vi "Update Array.vi"() -> ()   [LabVIEW 2013]
uses:
  Lockins.ctl
  Lockin.ctl
panel:
  in  "OSC used":i32
  in  "OSC Configuration":T1(array[cluster])
  out "Array":cluster{"Y":dbl[], "Y":dbl[]}[][](array[cluster])
  in  "Reset":bool=TRUE
  in  "Temperature":dbl
  in  "Lockins":T2 items=["Lock-in #1", "Lock-in #2", "Lock-in #3", "Lock-in #4"]
  in  "Results":dbl[][](array[numeric])
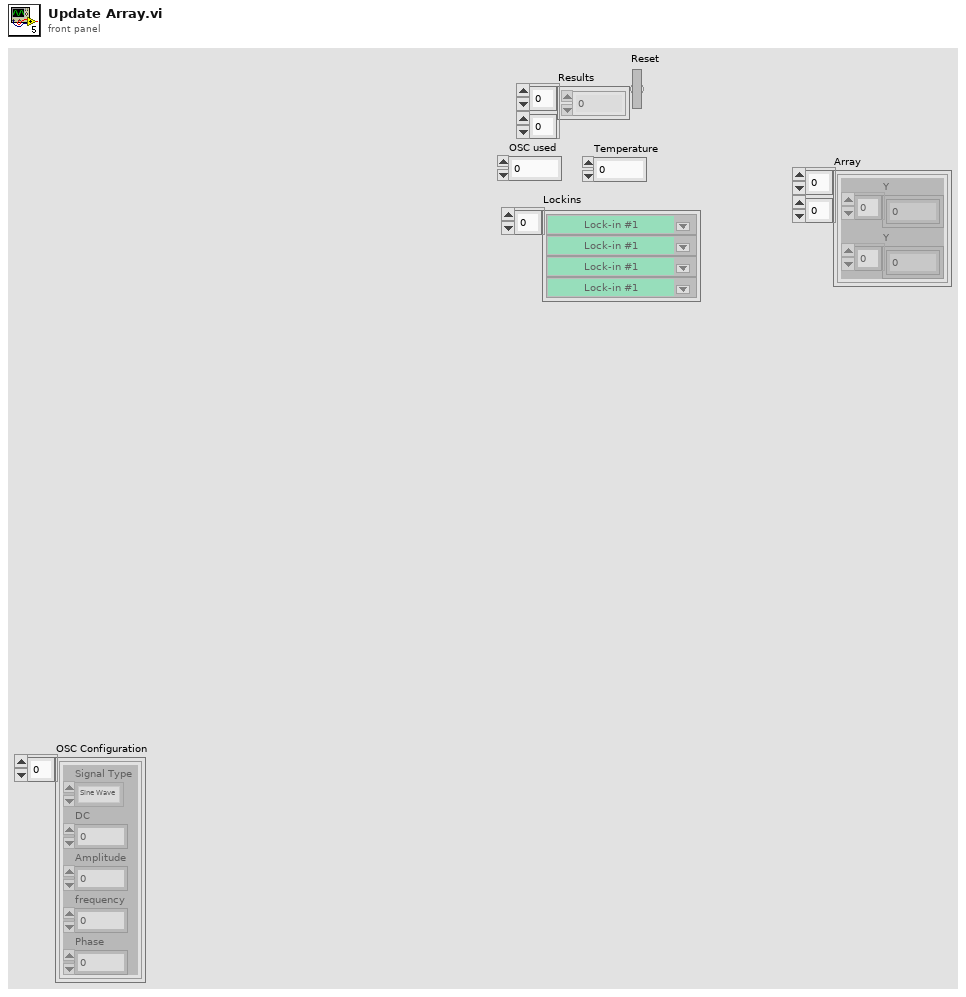
[diagram p1: front panel]
types:
  T1 = cluster{"Signal Type":enum16{"Sine Wave", "Triangle Wave", "Square Wave", "Sawtooth Wave"}, "DC":dbl, "Amplitude":dbl, "frequency":dbl, "Phase":dbl}[]
  T2 = typedef "Lockins.ctl" = T3[]
  T3 = typedef "Lockin.ctl" = u16
  T4 = cluster{"Signal Type":enum16{"Sine Wave", "Triangle Wave", "Square Wave", "Sawtooth Wave"}, "DC":dbl, "Amplitude":dbl, "frequency":dbl, "Phase":dbl}
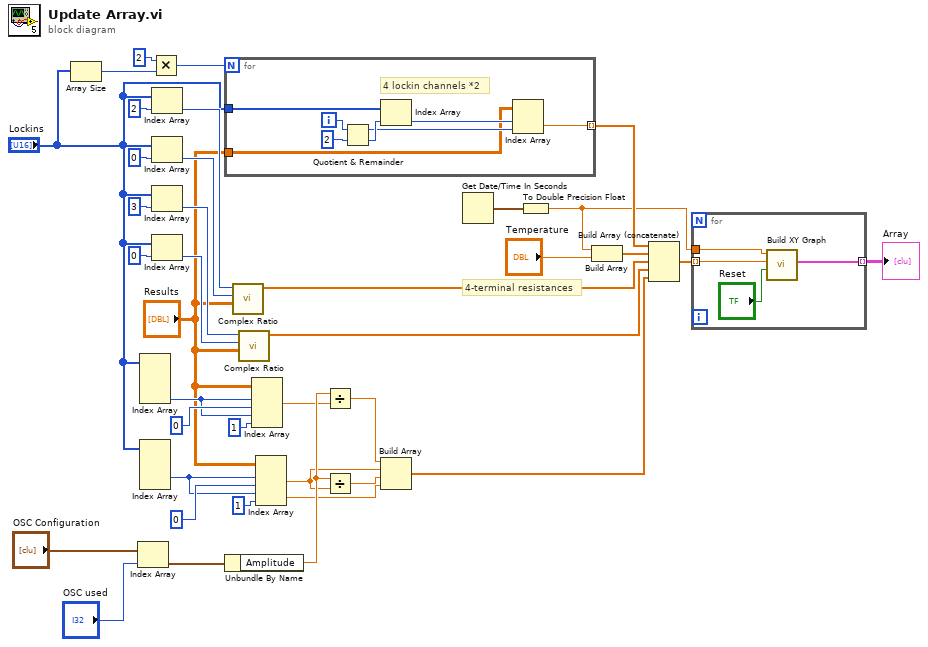
[diagram p0: block diagram]
diagram:
  # "4-terminal resistances"
  n1 = Array Size(array="Lockins") -> (size(s)=w37:i32)
  n2 = Index Array(array="OSC Configuration", index="OSC used") -> (element=w18:T4)
  n3 = Index Array(array="Lockins") -> (element #4=w13:T3)  [unwired: 4 in, 3 out]
  n4 = Index Array(array="Lockins") -> (element #3=w9:T3)  [unwired: 4 in, 3 out]
  n5 = Multiply(x=2, y=w37) -> (x*y=w36:i32)
  n6 = Index Array(array="Lockins", index=2) -> (element=w33:T3)
  n7 = Index Array(array="Lockins", index=0) -> (element=w32:T3)
  n8 = Index Array(array="Lockins", index=3) -> (element=w28:T3)
  n9 = Index Array(array="Lockins", index=0) -> (element=w29:T3)
  n10 = for {
    N: w36 -> [_]
    tunnel: "Lockins" -> [w42]
    tunnel: [w40] -> w27 mode=indexing
    tunnel: "Results" -> [w39]
    i -> [w45]
    # "4 lockin channels *2"
    n11 = Quotient & Remainder(x=w45, y=2) -> (x-y*floor(x/y)=w41:i32, floor(x/y)=w46:i32)
    n12 = Index Array(array=w42, index=w46) -> (element=w43:T3)
    n13 = Index Array(array=w39, index (row)=w43, index (col)=w41) -> (element=w40:dbl)
  }
  n14 = Unbundle By Name(w18) -> ("Amplitude"=w7:dbl)
  n15 = call "Complex Ratio.vi"("Results"="Results", "Lock-in denominator"=w32, "Lock-in numerator"=w33) -> ("Array"=w26:dbl[])  [unwired: 8 in]
  n16 = call "Complex Ratio.vi"("Results"="Results", "Lock-in denominator"=w29, "Lock-in numerator"=w28) -> ("Array"=w25:dbl[])  [unwired: 8 in]
  n17 = Index Array(array="Results", index (row) #1=w13, index (col) #1=0 ("disabled index (col)"), index (row) #2=w13, index (col) #2=1 ("disabled index (col)")) -> (element #1=w5:dbl)  [unwired: 1 out]
  n18 = Index Array(array="Results", index (row) #1=w9, index (col) #1=0 ("disabled index (col)"), index (row) #2=w9, index (col) #2=1 ("disabled index (col)")) -> (element #1=w2:dbl, element #2=w3:dbl)
  n19 = Divide(x=w7, y=w5) -> (x/y=w6:dbl)
  n20 = Divide(x=w7, y=w2) -> (x/y=w4:dbl)
  n21 = Build Array(w6, w2, w4, w3) -> (w1:dbl[])
  n22 = Get Date/Time In Seconds() -> (seconds since 1Jan1904=w24:timestamp)
  n23 = To Double Precision Float(number=w24) -> (double precision float=w21:dbl)
  n24 = Build Array(w21, "Temperature") -> (w22:dbl[])
  n25 = Build Array (concatenate)(w27, w22, w26, w25, w1) -> (w20:dbl[])
  n26 = for {
    tunnel: w21 -> [w50]
    tunnel: w20 -> [w49] mode=indexing
    tunnel: [w48] -> w19 mode=indexing
    n27 = call "Build XY Graph"("Reset"="Reset", "Y Input"=w49, "X Input"=w50) -> ("XY Graph"=w48:cluster{"Y":dbl[], "Y":dbl[]}[])  [unwired: 2 in, 6 out]
  }
  "Array" <- w19
